vi "CRYGraph Property Window Text.vi"(8 "Tab Name":string, 9 "Graph VI Ref":refnum<vi>) -> ()   [LabVIEW 2013]
uses:
  <vilib>/Utility/miscctls.llb/LVBoundsTypeDef.ctl
  CRYMainGlobal.vi
panel:
  out "Text":string
  in  "OK":bool
  in  "Text Tab":enum32{"Title", "Font"}(tab)
  in  "Title Name":string caption="标题名字"
  in  "Size":u32 caption="尺寸"
  in  "Plain":bool caption="纯文本"
  in  "Bold":bool caption="粗体"
  in  "Italic":bool caption="斜体"
  in  "Underline":bool caption="下划线"
  in  "Strikethrough":bool caption="删除线"
  in  "Color":u32(colorbox) caption="颜色"
  in  "Font":u16(ring) caption="字体" items=["Agency FB", "Agency FB Bold", "Aharoni Bold", "Algerian", "Andalus", "Angsana New", "Angsana New Bold", "Angsana New Bold Italic", "Angsana New Italic", "AngsanaUPC", "AngsanaUPC Bold", "AngsanaUPC Bold Italic", "AngsanaUPC Italic", "Aparajita", "Aparajita Bold", "Aparajita Bold Italic(TrueType)", "Aparajita Italic", "Arabic Typesetting", "Arial", "Arial Black", "Arial Bold", "Arial Bold Italic", "Arial Italic", "Arial Narrow", "Arial Narrow Bold", "Arial Narrow Bold Italic", "Arial Narrow Italic", "Arial Rounded MT Bold", "Arial Unicode MS", "Baskerville Old Face", "Batang & BatangChe & Gungsuh & GungsuhChe", "Bauhaus 93", "Bell MT", "Bell MT Bold", "Bell MT Italic", "Berlin Sans FB", "Berlin Sans FB Bold", "Berlin Sans FB Demi Bold", "Bernard MT Condensed", "Blackadder ITC", "Bodoni MT", "Bodoni MT Black", "Bodoni MT Black Italic", "Bodoni MT Bold", "Bodoni MT Bold Italic", "Bodoni MT Condensed", "Bodoni MT Condensed Bold", "Bodoni MT Condensed Bold Italic", "Bodoni MT Condensed Italic", "Bodoni MT Italic", "Bodoni MT Poster Compressed", "Book Antiqua", "Book Antiqua Bold", "Book Antiqua Bold Italic", "Book Antiqua Italic", "Bookman Old Style", "Bookman Old Style Bold", "Bookman Old Style Bold Italic", "Bookman Old Style Italic", "Bookshelf Symbol 7", "Bradley Hand ITC", "Britannic Bold", "Broadway", "Browallia New", "Browallia New Bold", "Browallia New Bold Italic", "Browallia New Italic", "BrowalliaUPC", "BrowalliaUPC Bold", "BrowalliaUPC Bold Italic", "BrowalliaUPC Italic", "Brush Script MT Italic", "Calibri", "Calibri Bold", "Calibri Bold Italic", "Calibri Italic", "Californian FB", "Californian FB Bold", "Californian FB Italic", "Calisto MT", "Calisto MT Bold", "Calisto MT Bold Italic", "Calisto MT Italic", "Cambria & Cambria Math", "Cambria Bold", "Cambria Bold Italic", "Cambria Italic", "Candara", "Candara Bold", "Candara Bold Italic", "Candara Italic", "Castellar", "Centaur", "Century", "Century Gothic", "Century Gothic Bold", "Century Gothic Bold Italic", "Century Gothic Italic", "Century Schoolbook", "Century Schoolbook Bold", "Century Schoolbook Bold Italic", "Century Schoolbook Italic", "Chiller", "Colonna MT", "Comic Sans MS", "Comic Sans MS Bold", "Consolas", "Consolas Bold", "Consolas Bold Italic", "Consolas Italic", "Constantia", "Constantia Bold", "Constantia Bold Italic", "Constantia Italic", "Cooper Black", "Copperplate Gothic Bold", "Copperplate Gothic Light", "Corbel", "Corbel Bold", "Corbel Bold Italic", "Corbel Italic", "Cordia New", "Cordia New Bold", "Cordia New Bold Italic", "Cordia New Italic", "CordiaUPC", "CordiaUPC Bold", "CordiaUPC Bold Italic", "CordiaUPC Italic", "Courier 10,12,15", "Courier New", "Courier New Bold", "Courier New Bold Italic", "Courier New Italic", "Curlz MT", "DFKai-SB", "DaunPenh", "David", "David Bold", "DilleniaUPC", "DilleniaUPC Bold", "DilleniaUPC Bold Italic", "DilleniaUPC Italic", "DokChampa", "Ebrima", "Ebrima Bold", "Edwardian Script ITC", "Elephant", "Elephant Italic", "Engravers MT", "Eras Bold ITC", "Eras Demi ITC", "Eras Light ITC", "Eras Medium ITC", "Estrangelo Edessa", "EucrosiaUPC", "EucrosiaUPC Bold", "EucrosiaUPC Bold Italic", "EucrosiaUPC Italic", "Euphemia", "FangSong", "Felix Titling", "Footlight MT Light", "Forte", "FrankRuehl", "Franklin Gothic Book", "Franklin Gothic Book Italic", "Franklin Gothic Demi", "Franklin Gothic Demi Cond", "Franklin Gothic Demi Italic", "Franklin Gothic Heavy", "Franklin Gothic Heavy Italic", "Franklin Gothic Medium", "Franklin Gothic Medium Cond", "Franklin Gothic Medium Italic", "FreesiaUPC", "FreesiaUPC Bold", "FreesiaUPC Bold Italic", "FreesiaUPC Italic", "Freestyle Script", "French Script MT", "Gabriola", "Garamond", "Garamond Bold", "Garamond Italic", "Gautami", "Gautami Bold", "Georgia", "Georgia Bold", "Georgia Bold Italic", "Georgia Italic", "Gigi", "Gill Sans MT", "Gill Sans MT Bold", "Gill Sans MT Bold Italic", "Gill Sans MT Condensed", "Gill Sans MT Ext Condensed Bold", "Gill Sans MT Italic", "Gill Sans Ultra Bold", "Gill Sans Ultra Bold Condensed", "Gisha", "Gisha Bold", "Gloucester MT Extra Condensed", "Goudy Old Style", "Goudy Old Style Bold", "Goudy Old Style Italic", "Goudy Stout", "Gulim & GulimChe & Dotum & DotumChe", "Haettenschweiler", "Harlow Solid Italic", "Harrington", "High Tower Text", "High Tower Text Italic", "Impact", "Imprint MT Shadow", "Informal Roman", "IrisUPC", "IrisUPC Bold", "IrisUPC Bold Italic", "IrisUPC Italic", "Iskoola Pota", "Iskoola Pota Bold", "JasmineUPC", "JasmineUPC Bold", "JasmineUPC Bold Italic", "JasmineUPC Italic", "Jokerman", "Juice ITC", "KaiTi", "Kalinga", "Kalinga Bold", "Kartika", "Kartika Bold", "Khmer UI", "Khmer UI Bold", "KodchiangUPC", "KodchiangUPC Bold", "KodchiangUPC Bold Italic", "KodchiangUPC Italic", "Kokila", "Kokila Bold", "Kokila Bold Italic(TrueType)", "Kokila Italic", "Kristen ITC", "Kunstler Script", "Lao UI", "Lao UI Bold", "Latha", "Latha Bold", "Leelawadee", "Leelawadee Bold", "Levenim MT", "Levenim MT Bold", "LilyUPC", "LilyUPC Bold", "LilyUPC Bold Italic", "LilyUPC Italic", "Lucida Bright", "Lucida Bright Demibold", "Lucida Bright Demibold Italic", "Lucida Bright Italic", "Lucida Calligraphy Italic", "Lucida Console", "Lucida Fax Demibold", "Lucida Fax Demibold Italic", "Lucida Fax Italic", "Lucida Fax Regular", "Lucida Handwriting Italic", "Lucida Sans Demibold Italic", "Lucida Sans Demibold Roman", "Lucida Sans Italic", "Lucida Sans Regular", "Lucida Sans Typewriter Bold", "Lucida Sans Typewriter Bold Oblique", "Lucida Sans Typewriter Oblique", "Lucida Sans Typewriter Regular", "Lucida Sans Unicode", "MS Gothic & MS PGothic & MS UI Gothic", "MS Mincho", "MS Mincho & MS PMincho", "MS Outlook", "MS Reference Sans Serif", "MS Reference Specialty", "MS Sans Serif 8,10,12,14,18,24", "MS Serif 8,10,12,14,18,24", "MT Extra", "MV Boli", "Magneto Bold", "Maiandra GD", "Malgun Gothic", "Malgun Gothic Bold", "Mangal", "Mangal Bold", "Matura MT Script Capitals", "Meiryo & Meiryo Italic & Meiryo UI & Meiryo UI Italic", "Meiryo Bold & Meiryo Bold Italic & Meiryo UI Bold & Meiryo UI Bold Italic", "Microsoft Himalaya", "Microsoft JhengHei", "Microsoft JhengHei Bold", "Microsoft New Tai Lue", "Microsoft New Tai Lue Bold", "Microsoft PhagsPa", "Microsoft PhagsPa Bold", "Microsoft Sans Serif", "Microsoft Tai Le", "Microsoft Tai Le Bold", "Microsoft Uighur", "Microsoft YaHei", "Microsoft YaHei Bold", "Microsoft Yi Baiti", "MingLiU & PMingLiU & MingLiU_HKSCS", "MingLiU-ExtB & PMingLiU-ExtB & MingLiU_HKSCS-ExtB", "Miriam", "Miriam Fixed", "Mistral", "Modern", "Modern No. 20", "Mongolian Baiti", "Monotype Corsiva", "MoolBoran", "Narkisim", "Niagara Engraved", "Niagara Solid", "Nyala", "OCR A Extended", "Old English Text MT", "Onyx", "Palace Script MT", "Palatino Linotype", "Palatino Linotype Bold", "Palatino Linotype Bold Italic", "Palatino Linotype Italic", "Papyrus", "Parchment", "Perpetua", "Perpetua Bold", "Perpetua Bold Italic", "Perpetua Italic", "Perpetua Titling MT Bold", "Perpetua Titling MT Light", "Plantagenet Cherokee", "Playbill", "Poor Richard", "Pristina", "Raavi", "Raavi Bold", "Rage Italic", "Ravie", "Rockwell", "Rockwell Bold", "Rockwell Bold Italic", "Rockwell Condensed", "Rockwell Condensed Bold", "Rockwell Extra Bold", "Rockwell Italic", "Rod", "Roman", "Sakkal Majalla", "Sakkal Majalla Bold", "Script", "Script MT Bold", "Segoe Print", "Segoe Print Bold", "Segoe Script", "Segoe Script Bold", "Segoe UI", "Segoe UI Bold", "Segoe UI Bold Italic", "Segoe UI Italic", "Segoe UI Light", "Segoe UI Semibold", "Segoe UI Symbol", "Shonar Bangla", "Shonar Bangla Bold", "Showcard Gothic", "Shruti", "Shruti Bold", "SimHei", "SimSun & NSimSun", "SimSun-ExtB", "Simplified Arabic", "Simplified Arabic Bold", "Simplified Arabic Fixed", "Small Fonts", "Small Fonts", "Snap ITC", "Stencil", "Sylfaen", "Symbol", "Tahoma", "Tahoma Bold", "Tempus Sans ITC", "Tera Special", "Times New Roman", "Times New Roman Bold", "Times New Roman Bold Italic", "Times New Roman Italic", "Traditional Arabic", "Traditional Arabic Bold", "Trebuchet MS", "Trebuchet MS Bold", "Trebuchet MS Bold Italic", "Trebuchet MS Italic", "Tunga", "Tunga Bold", "Tw Cen MT", "Tw Cen MT Bold", "Tw Cen MT Bold Italic", "Tw Cen MT Condensed", "Tw Cen MT Condensed Bold", "Tw Cen MT Condensed Extra Bold", "Tw Cen MT Italic", "Utsaah", "Utsaah Bold", "Utsaah Bold Italic(TrueType)", "Utsaah Italic", "Vani", "Vani Bold", "Verdana", "Verdana Bold", "Verdana Bold Italic", "Verdana Italic", "Vijaya", "Vijaya Bold", "Viner Hand ITC", "Vivaldi Italic", "Vladimir Script", "Vrinda", "Vrinda Bold", "Webdings", "Wide Latin", "Wingdings", "Wingdings 2", "Wingdings 3"]
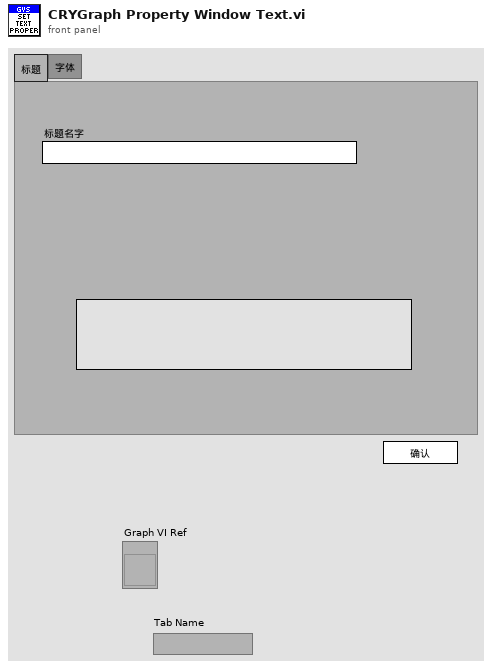
[diagram p1: front panel]
types:
  T1 = enum32{"English", "Chinese", "Korean", "Japanese", "Russian", "Chinese traditional"}
  T2 = typedef "LVBoundsTypeDef.ctl" = cluster{"Width":u32, "Height":u32}
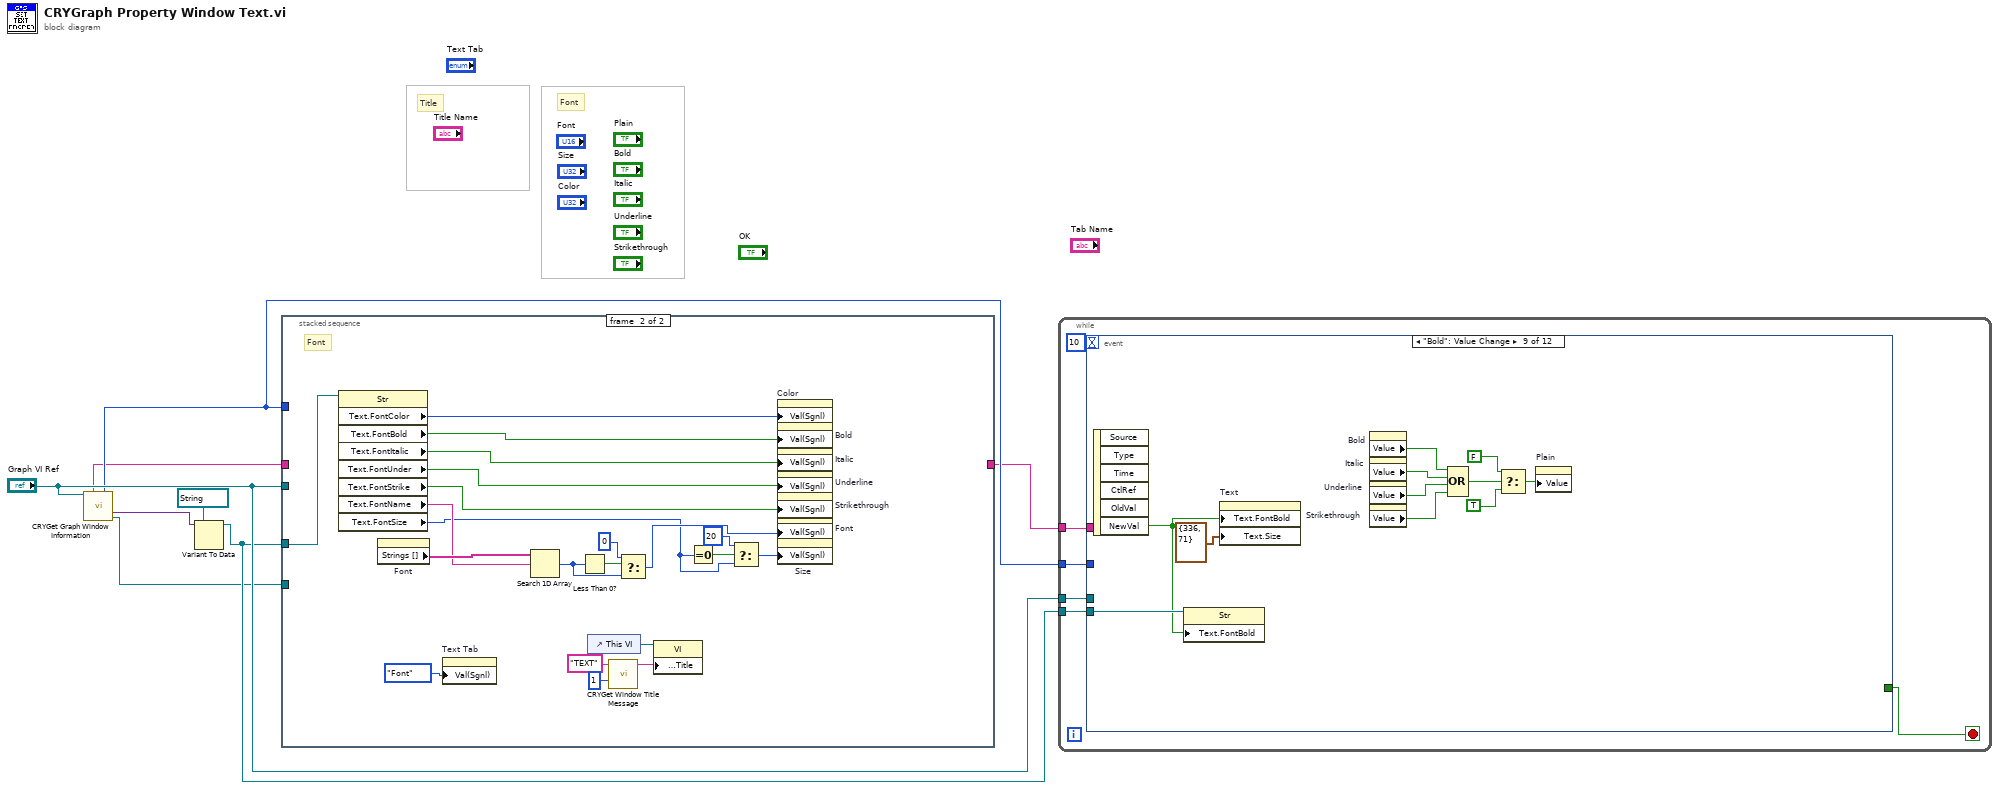
[diagram p0: block diagram]
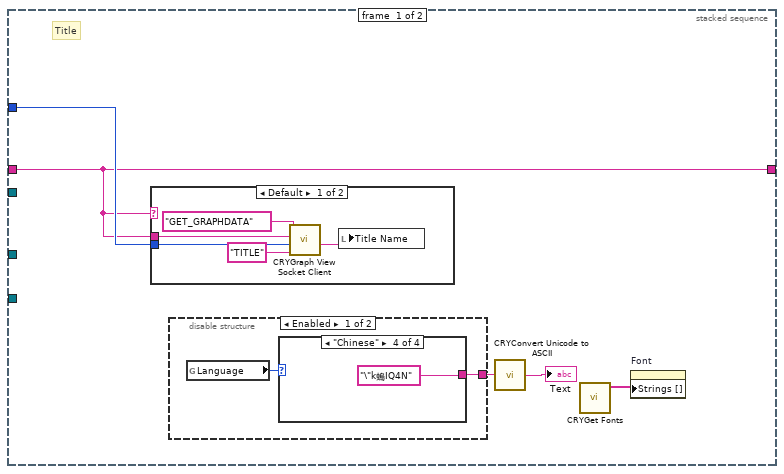
[diagram p2: hidden frame]
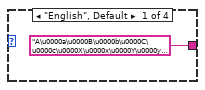
[diagram p3: hidden frame]
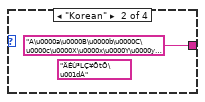
[diagram p4: hidden frame]
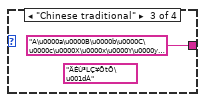
[diagram p5: hidden frame]
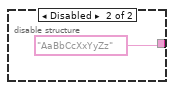
[diagram p6: hidden frame]
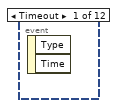
[diagram p8: hidden frame]
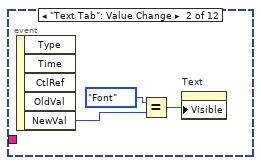
[diagram p9: hidden frame]
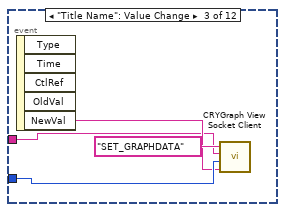
[diagram p10: hidden frame]
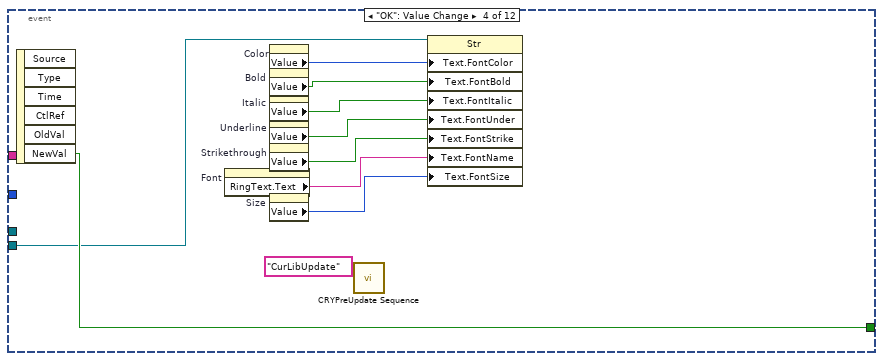
[diagram p11: hidden frame]
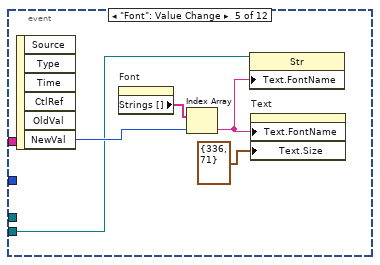
[diagram p12: hidden frame]
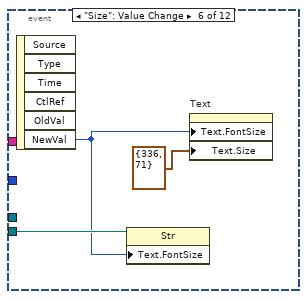
[diagram p13: hidden frame]
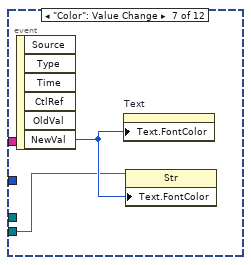
[diagram p14: hidden frame]
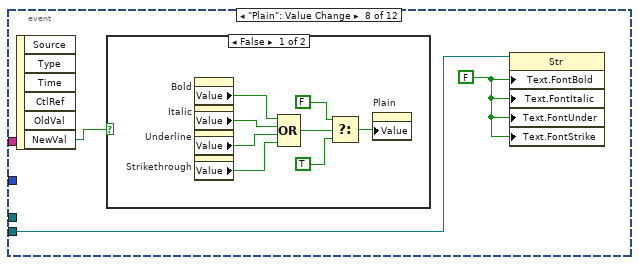
[diagram p15: hidden frame]
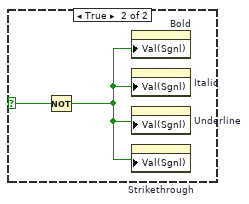
[diagram p16: hidden frame]
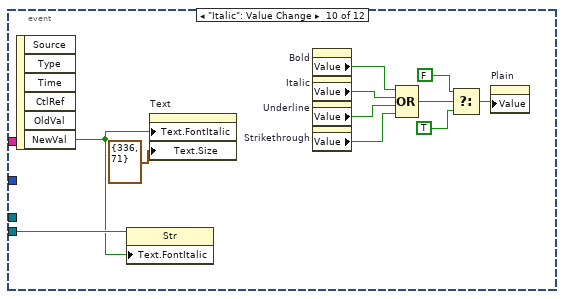
[diagram p17: hidden frame]
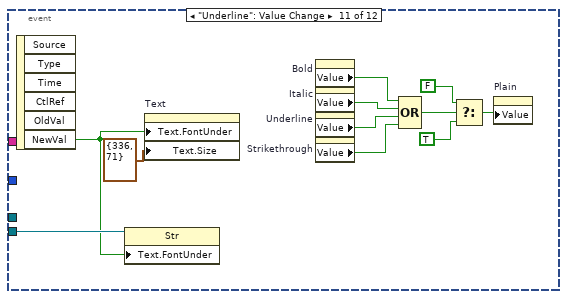
[diagram p18: hidden frame]
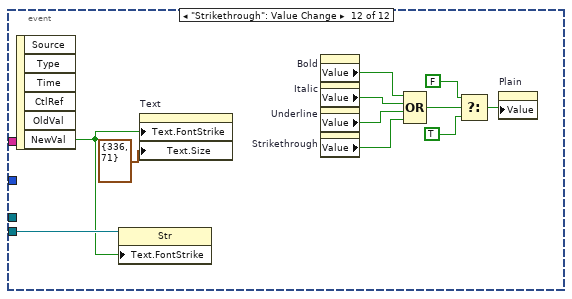
[diagram p19: hidden frame]
diagram:
  # "Title"
  # "Font"
  n1 = call "CRYGet Graph Window Information.vi"("pGraph VI In"="Graph VI Ref") -> ("Queue Name Out"=w4:string, "Graph Number Out"=w5:i32, "Graph Control Ref Out"=w1:variant, "Legend Ref Out"=w6:refnum<vi>)  [unwired: 2 in, 9 out]
  n2 = Variant To Data(type=refnum<vi> refnum ("Graph Ref"), Variant=w1) -> (data=w7:refnum<vi>)  [unwired: 1 in, 1 out]
  n3 = stacked-sequence {
    tunnel: "Graph VI Ref" -> [_ _]
    tunnel: w7 -> [_ w38]
    tunnel: w6 -> [_ _]
    tunnel: w5 -> [w12 _]
    tunnel: w4 -> [w11 _]
    tunnel: [w11 _] -> w3
    frame #0 {
      # "Title"
      n4 = case shown="Default" w11 {
        tunnel: w12 -> [w23 _]
        tunnel: w11 -> [w21 _]
        frame Default {
          n5 = call "CRYGraph View Socket Client.vi"("sOption"="TITLE", "nData"=w23, "sData"=w21, "sAction"="GET_GRAPHDATA") -> ("sData Out"=w22:string)  [unwired: 4 in, 3 out]
          n6 = local write "Title Name"(w22) -> ()
        }
        frame "test DataView" {
        }
      }
      n7 = disable-structure shown="Enabled" {
        disable-tunnel: [w15 "AaBbCcXxYyZz" ("WaterMarkText")] -> w10
        frame Enabled {
          n8 = global read "CRYMainGlobal.vi" "Language"() -> (w14:T1)
          n9 = case shown="\"Chinese\"" w14 {
            tunnel: ["A\u0000a\u0000B\u0000b\u0000C\u0000c\u0000X\u0000x\u0000Y\u0000y\u0000Z\u0000z\u0000" ("WaterMarkText") "A\u0000a\u0000B\u0000b\u0000C\u0000c\u0000X\u0000x\u0000Y\u0000y\u0000Z\u0000z\u0000" ("Unicode String") "A\u0000a\u0000B\u0000b\u0000C\u0000c\u0000X\u0000x\u0000Y\u0000y\u0000Z\u0000z\u0000" ("Unicode String") "\"k螐IQ4N" ("Unicode String")] -> w15
            frame "English", Default {
            }
            frame "Korean" {
              (unwired) "ÄÉÙ³LÇ¥ÕtÕ\u001dÁ" ("Unicode String")
            }
            frame "Chinese traditional" {
              (unwired) "ÄÉÙ³LÇ¥ÕtÕ\u001dÁ" ("Unicode String")
            }
            frame "Chinese" {
            }
          }
        }
        frame Disabled {
        }
      }
      n10 = call "CRYConvert Unicode to ASCII.vi"("Unicode"=w10) -> ("ASCII"=→"Text":string)  [unwired: 4 in]
      n11 = call "CRYGet Fonts.vi"() -> ("Fonts out"=w13:string[])  [unwired: 11 out]
      n12 = property on="Font" class="Ring (strict)"("Strings []"=w13) -> ()  [unwired: 2 in, 2 out]
    }
    frame #1 {
      # "Font"
      n13 = property class="Str"(reference=w38) -> ("Text.FontColor"=w37:u32, "Text.FontBold"=w36:bool, "Text.FontItalic"=w35:bool, "Text.FontUnder"=w34:bool, "Text.FontStrike"=w33:bool, "Text.FontName"=w32:string, "Text.FontSize"=w31:u32)  [unwired: 1 in, 2 out]
      n14 = property on="Font" class="Ring (strict)"() -> ("Strings []"=w43:string[])  [unwired: 2 in, 2 out]
      n15 = property on="Text Tab" class="TabCtl (strict)"("Val(Sgnl)"=enum32{"Title", "Font"}."Font" ("Text Tab")) -> ()  [unwired: 2 in, 2 out]
      n16 = Search 1D Array(1D array=w43, element=w32) -> (index of element=w40:i32)  [unwired: 1 out]
      n17 = Less Than 0?(x=w40) -> (x < 0?=w42:bool)
      n18 = control-ref of="This VI"() -> (w27:refnum<vi>)
      n19 = call "CRYGet Window Title Message.vi"("No"=1 ("Error No"), "Kind"="TEXT") -> ("Multibyte String"=w28:string)  [unwired: 4 in, 5 out]
      n20 = Select(t=u32 0 ("Value (Signaling)"), s=w42, f=w40) -> (s? t:f=w39:u32)
      n21 = property class="VI"(reference=w27, "Front Panel.Title"=w28) -> ()  [unwired: 1 in, 2 out]
      n22 = Equal To 0?(x=w31) -> (x = 0?=w46:bool)
      n23 = Select(t=u32 20 ("Value (Signaling)"), s=w46, f=w31) -> (s? t:f=w44:u32)
      n24 = property on="Color" class="ColBox"("Val(Sgnl)"=w37) -> ()  [unwired: 2 in, 2 out]
      n25 = property on="Bold" class="Bool (strict)"("Val(Sgnl)"=w36) -> ()  [unwired: 2 in, 2 out]
      n26 = property on="Italic" class="Bool (strict)"("Val(Sgnl)"=w35) -> ()  [unwired: 2 in, 2 out]
      n27 = property on="Underline" class="Bool (strict)"("Val(Sgnl)"=w34) -> ()  [unwired: 2 in, 2 out]
      n28 = property on="Strikethrough" class="Bool (strict)"("Val(Sgnl)"=w33) -> ()  [unwired: 2 in, 2 out]
      n29 = property on="Font" class="Ring (strict)"("Val(Sgnl)"=w39) -> ()  [unwired: 2 in, 2 out]
      n30 = property on="Size" class="DigNum (strict)"("Val(Sgnl)"=w44) -> ()  [unwired: 2 in, 2 out]
    }
  }
  n31 = while {
    tunnel: "Graph VI Ref" -> [w51]
    tunnel: w7 -> [w50]
    tunnel: w5 -> [w48]
    tunnel: w3 -> [w47]
    stop <- w49 stop-if-true
    n32 = event shown="[8] \"Bold\": Value Change" {
      selector: _ -> [_ _ _ _ _ _ _ _ _ _ _ _]
      dyn-events: _ -> [_ _ _ _ _ _ _ _ _ _ _ _]
      timeout: 10 -> [_ _ _ _ _ _ _ _ _ _ _ _]
      tunnel: [_ _ _ w69 _ _ _ _ _ _ _ _] -> w49
      tunnel: w51 -> [_ _ _ _ _ _ _ _ _ _ _ _]
      tunnel: w50 -> [_ _ _ w68 w72 w77 w78 w81 w95 w106 w117 w128]
      tunnel: w48 -> [_ _ w58 _ _ _ _ _ _ _ _ _]
      tunnel: w47 -> [_ _ w56 _ _ _ _ _ _ _ _ _]
      event Timeout {
        n33 = event-data() -> ()  [unwired: 3 out]
      }
      event "Text Tab": Value Change {
        n34 = event-data() -> ("NewVal"=w54:enum32{"Title", "Font"})  [unwired: 5 out]
        n35 = Equal?(x=enum32{"Title", "Font"}."Font" ("NewVal"), y=w54) -> (x = y?=w53:bool)
        n36 = property on="Text" class="Str"("Visible"=w53) -> ()  [unwired: 2 in, 2 out]
      }
      event "Title Name": Value Change {
        n37 = event-data() -> ("NewVal"=w57:string)  [unwired: 5 out]
        n38 = call "CRYGraph View Socket Client.vi"("sOption"=w57, "nData"=w58, "sData"=w56, "sAction"="SET_GRAPHDATA") -> ()  [unwired: 4 in, 4 out]
      }
      event "OK": Value Change {
        n39 = event-data() -> ("NewVal"=w69:bool)  [unwired: 6 out]
        n40 = property on="Font" class="Ring (strict)"() -> ("RingText.Text"=w62:string)  [unwired: 2 in, 2 out]
        n41 = property on="Color" class="ColBox"() -> ("Value"=w67:u32)  [unwired: 2 in, 2 out]
        n42 = property on="Bold" class="Bool (strict)"() -> ("Value"=w66:bool)  [unwired: 2 in, 2 out]
        n43 = property on="Italic" class="Bool (strict)"() -> ("Value"=w65:bool)  [unwired: 2 in, 2 out]
        n44 = property on="Underline" class="Bool (strict)"() -> ("Value"=w64:bool)  [unwired: 2 in, 2 out]
        n45 = property on="Strikethrough" class="Bool (strict)"() -> ("Value"=w63:bool)  [unwired: 2 in, 2 out]
        n46 = property on="Size" class="DigNum (strict)"() -> ("Value"=w61:u32)  [unwired: 2 in, 2 out]
        n47 = call "CRYPreUpdate Sequence.vi"("EventName"="CurLibUpdate") -> ()  [unwired: 15 in]
        n48 = property class="Str"(reference=w68, "Text.FontColor"=w67, "Text.FontBold"=w66, "Text.FontItalic"=w65, "Text.FontUnder"=w64, "Text.FontStrike"=w63, "Text.FontName"=w62, "Text.FontSize"=w61) -> ()  [unwired: 1 in, 2 out]
      }
      event "Font": Value Change {
        n49 = event-data() -> ("NewVal"=w74:u16)  [unwired: 6 out]
        n50 = property on="Font" class="Ring (strict)"() -> ("Strings []"=w73:string[])  [unwired: 2 in, 2 out]
        n51 = Index Array(array=w73, index=w74) -> (element=w71:string)
        n52 = property class="Str"(reference=w72, "Text.FontName"=w71) -> ()  [unwired: 1 in, 2 out]
        n53 = property on="Text" class="Str"("Text.FontName"=w71, "Text.Size"=T2 {"Width"=336, "Height"=71}) -> ()  [unwired: 2 in, 2 out]
      }
      event "Size": Value Change {
        n54 = event-data() -> ("NewVal"=w76:u32)  [unwired: 6 out]
        n55 = property class="Str"(reference=w77, "Text.FontSize"=w76) -> ()  [unwired: 1 in, 2 out]
        n56 = property on="Text" class="Str"("Text.FontSize"=w76, "Text.Size"=T2 {"Width"=336, "Height"=71}) -> ()  [unwired: 2 in, 2 out]
      }
      event "Color": Value Change {
        n57 = event-data() -> ("NewVal"=w79:u32)  [unwired: 6 out]
        n58 = property on="Text" class="Str"("Text.FontColor"=w79) -> ()  [unwired: 2 in, 2 out]
        n59 = property class="Str"(reference=w78, "Text.FontColor"=w79) -> ()  [unwired: 1 in, 2 out]
      }
      event "Plain": Value Change {
        w80 = FALSE ("Text.Font:Bold")
        n60 = event-data() -> ("NewVal"=w82:bool)  [unwired: 6 out]
        n61 = case shown="False" w82 {
          selector: w82 -> [_ w92]
          frame False {
            n62 = property on="Bold" class="Bool (strict)"() -> ("Value"=w87:bool)  [unwired: 2 in, 2 out]
            n63 = property on="Italic" class="Bool (strict)"() -> ("Value"=w88:bool)  [unwired: 2 in, 2 out]
            n64 = property on="Underline" class="Bool (strict)"() -> ("Value"=w89:bool)  [unwired: 2 in, 2 out]
            n65 = property on="Strikethrough" class="Bool (strict)"() -> ("Value"=w90:bool)  [unwired: 2 in, 2 out]
            n66 = Compound Arithmetic op=OR(w87, w88, w89, w90) -> (w86:bool)
            n67 = Select(t=FALSE, s=w86, f=TRUE) -> (s? t:f=w83:bool)
            n68 = property on="Plain" class="Bool (strict)"("Value"=w83) -> ()  [unwired: 2 in, 2 out]
          }
          frame True {
            n69 = Not(x=w92) -> (.not. x?=w91:bool)
            n70 = property on="Bold" class="Bool (strict)"("Val(Sgnl)"=w91) -> ()  [unwired: 2 in, 2 out]
            n71 = property on="Italic" class="Bool (strict)"("Val(Sgnl)"=w91) -> ()  [unwired: 2 in, 2 out]
            n72 = property on="Underline" class="Bool (strict)"("Val(Sgnl)"=w91) -> ()  [unwired: 2 in, 2 out]
            n73 = property on="Strikethrough" class="Bool (strict)"("Val(Sgnl)"=w91) -> ()  [unwired: 2 in, 2 out]
          }
        }
        n74 = property class="Str"(reference=w81, "Text.FontBold"=w80, "Text.FontItalic"=w80, "Text.FontUnder"=w80, "Text.FontStrike"=w80) -> ()  [unwired: 1 in, 2 out]
      }
      event "Bold": Value Change {
        n75 = event-data() -> ("NewVal"=w94:bool)  [unwired: 6 out]
        n76 = property class="Str"(reference=w95, "Text.FontBold"=w94) -> ()  [unwired: 1 in, 2 out]
        n77 = property on="Text" class="Str"("Text.FontBold"=w94, "Text.Size"=T2 {"Width"=336, "Height"=71}) -> ()  [unwired: 2 in, 2 out]
        n78 = property on="Bold" class="Bool (strict)"() -> ("Value"=w96:bool)  [unwired: 2 in, 2 out]
        n79 = property on="Italic" class="Bool (strict)"() -> ("Value"=w97:bool)  [unwired: 2 in, 2 out]
        n80 = property on="Underline" class="Bool (strict)"() -> ("Value"=w98:bool)  [unwired: 2 in, 2 out]
        n81 = property on="Strikethrough" class="Bool (strict)"() -> ("Value"=w99:bool)  [unwired: 2 in, 2 out]
        n82 = Compound Arithmetic op=OR(w96, w97, w98, w99) -> (w100:bool)
        n83 = Select(t=FALSE, s=w100, f=TRUE) -> (s? t:f=w103:bool)
        n84 = property on="Plain" class="Bool (strict)"("Value"=w103) -> ()  [unwired: 2 in, 2 out]
      }
      event "Italic": Value Change {
        n85 = event-data() -> ("NewVal"=w105:bool)  [unwired: 6 out]
        n86 = property class="Str"(reference=w106, "Text.FontItalic"=w105) -> ()  [unwired: 1 in, 2 out]
        n87 = property on="Text" class="Str"("Text.FontItalic"=w105, "Text.Size"=T2 {"Width"=336, "Height"=71}) -> ()  [unwired: 2 in, 2 out]
        n88 = property on="Bold" class="Bool (strict)"() -> ("Value"=w107:bool)  [unwired: 2 in, 2 out]
        n89 = property on="Italic" class="Bool (strict)"() -> ("Value"=w108:bool)  [unwired: 2 in, 2 out]
        n90 = property on="Underline" class="Bool (strict)"() -> ("Value"=w109:bool)  [unwired: 2 in, 2 out]
        n91 = property on="Strikethrough" class="Bool (strict)"() -> ("Value"=w110:bool)  [unwired: 2 in, 2 out]
        n92 = Compound Arithmetic op=OR(w107, w108, w109, w110) -> (w111:bool)
        n93 = Select(t=FALSE, s=w111, f=TRUE) -> (s? t:f=w114:bool)
        n94 = property on="Plain" class="Bool (strict)"("Value"=w114) -> ()  [unwired: 2 in, 2 out]
      }
      event "Underline": Value Change {
        n95 = event-data() -> ("NewVal"=w116:bool)  [unwired: 6 out]
        n96 = property class="Str"(reference=w117, "Text.FontUnder"=w116) -> ()  [unwired: 1 in, 2 out]
        n97 = property on="Text" class="Str"("Text.FontUnder"=w116, "Text.Size"=T2 {"Width"=336, "Height"=71}) -> ()  [unwired: 2 in, 2 out]
        n98 = property on="Bold" class="Bool (strict)"() -> ("Value"=w118:bool)  [unwired: 2 in, 2 out]
        n99 = property on="Italic" class="Bool (strict)"() -> ("Value"=w119:bool)  [unwired: 2 in, 2 out]
        n100 = property on="Underline" class="Bool (strict)"() -> ("Value"=w120:bool)  [unwired: 2 in, 2 out]
        n101 = property on="Strikethrough" class="Bool (strict)"() -> ("Value"=w121:bool)  [unwired: 2 in, 2 out]
        n102 = Compound Arithmetic op=OR(w118, w119, w120, w121) -> (w122:bool)
        n103 = Select(t=FALSE, s=w122, f=TRUE) -> (s? t:f=w125:bool)
        n104 = property on="Plain" class="Bool (strict)"("Value"=w125) -> ()  [unwired: 2 in, 2 out]
      }
      event "Strikethrough": Value Change {
        n105 = event-data() -> ("NewVal"=w127:bool)  [unwired: 6 out]
        n106 = property class="Str"(reference=w128, "Text.FontStrike"=w127) -> ()  [unwired: 1 in, 2 out]
        n107 = property on="Text" class="Str"("Text.FontStrike"=w127, "Text.Size"=T2 {"Width"=336, "Height"=71}) -> ()  [unwired: 2 in, 2 out]
        n108 = property on="Bold" class="Bool (strict)"() -> ("Value"=w129:bool)  [unwired: 2 in, 2 out]
        n109 = property on="Italic" class="Bool (strict)"() -> ("Value"=w130:bool)  [unwired: 2 in, 2 out]
        n110 = property on="Underline" class="Bool (strict)"() -> ("Value"=w131:bool)  [unwired: 2 in, 2 out]
        n111 = property on="Strikethrough" class="Bool (strict)"() -> ("Value"=w132:bool)  [unwired: 2 in, 2 out]
        n112 = Compound Arithmetic op=OR(w129, w130, w131, w132) -> (w133:bool)
        n113 = Select(t=FALSE, s=w133, f=TRUE) -> (s? t:f=w136:bool)
        n114 = property on="Plain" class="Bool (strict)"("Value"=w136) -> ()  [unwired: 2 in, 2 out]
      }
    }
  }
